vi "value updation while typing.vi"() -> ()   [LabVIEW 2025]
panel:
  out "output String 2":string
  in  "input String":string
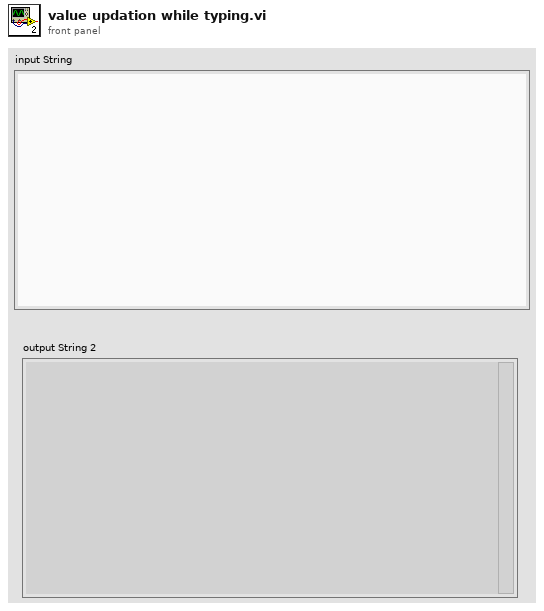
[diagram p1: front panel]
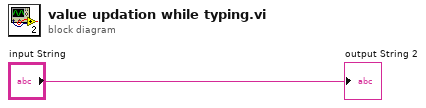
[diagram p0: block diagram]
diagram:
  "output String 2" <- "input String"
